vi "specu1a 1.0.0 PInfo Cluster to PInfo String.vi"(1 "output cluster":T2={"UnitID"={0, 0, 0, 0, 0, 0, 0, 0}, "Sensor Name"={0, 0, 0, 0, 0, 0, 0, 0, 0, 0, 0, 0, 0, 0, 0, 0}, "Serial Number"={0, 0, 0, 0, 0, 0, 0, 0}, "Reserved"={0, 0, 0, 0, 0, 0, 0, 0}, "Wave Upper"=630, "Wave Lower"=1050}) -> (0 "output cluster 2":T1={"UnitID"="", "Sensor Name"="", "Serial Number"="", "Reserved"="", "Wave Upper"=630, "Wave Lower"=1050})   [LabVIEW 2019]
uses:
  Controls/specu1a 1.0.0 Product Information.ctl
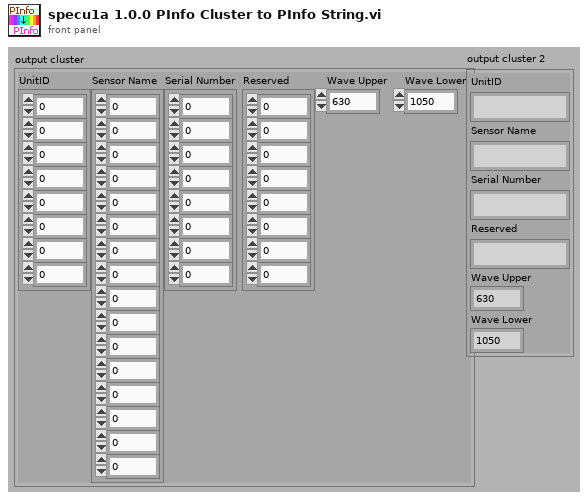
[diagram p1: front panel]
types:
  T1 = typedef "specu1a 1.0.0 Product Information.ctl" = cluster{"UnitID":string, "Sensor Name":string, "Serial Number":string, "Reserved":string, "Wave Upper":u16, "Wave Lower":u16}
  T2 = cluster{"UnitID":cluster{u8, u8, u8, u8, u8, u8, u8, u8}, "Sensor Name":cluster{u8, u8, u8, u8, u8, u8, u8, u8, u8, u8, u8, u8, u8, u8, u8, u8}, "Serial Number":cluster{u8, u8, u8, u8, u8, u8, u8, u8}, "Reserved":cluster{u8, u8, u8, u8, u8, u8, u8, u8}, "Wave Upper":u16, "Wave Lower":u16}
  T3 = cluster{u8, u8, u8, u8, u8, u8, u8, u8, u8, u8, u8, u8, u8, u8, u8, u8}
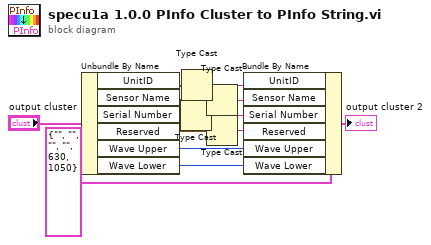
[diagram p0: block diagram]
diagram:
  n1 = Unbundle By Name("output cluster") -> ("UnitID"=w12:cluster{u8, u8, u8, u8, u8, u8, u8, u8}, "Sensor Name"=w11:T3, "Serial Number"=w10:cluster{u8, u8, u8, u8, u8, u8, u8, u8}, "Reserved"=w9:cluster{u8, u8, u8, u8, u8, u8, u8, u8}, "Wave Upper"=w7:u16, "Wave Lower"=w8:u16)
  n2 = Type Cast(x=w10) -> (*(type *) &x=w5:string)  [unwired: 1 in]
  n3 = Type Cast(x=w12) -> (*(type *) &x=w3:string)  [unwired: 1 in]
  n4 = Type Cast(x=w11) -> (*(type *) &x=w4:string)  [unwired: 1 in]
  n5 = Type Cast(x=w9) -> (*(type *) &x=w6:string)  [unwired: 1 in]
  n6 = Bundle By Name(cluster=T1 {"UnitID"="", "Sensor Name"="", "Serial Number"="", "Reserved"="", "Wave Upper"=630, "Wave Lower"=1050} ("Unit Information"), "UnitID"=w3, "Sensor Name"=w4, "Serial Number"=w5, "Reserved"=w6, "Wave Upper"=w7, "Wave Lower"=w8) -> (→"output cluster 2":T1)
